vi "Create Reference.vi"(8 "error in (no error)":errorcluster, 11 "Generic":refnum<class "Generic.lvclass">) -> (0 "error out":errorcluster, 3 "Generic Reference":refnum<data-value>)   [LabVIEW 2013, in "Hierarchy Framework.lvlib" / "Generic.lvclass"]
doc: "Create class object data value reference."
uses:
  Generic.lvclass
panel:
  out "Generic Reference":u64
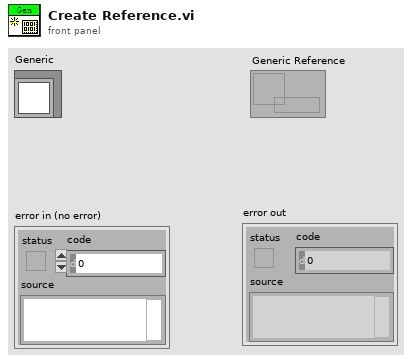
[diagram p1: front panel]
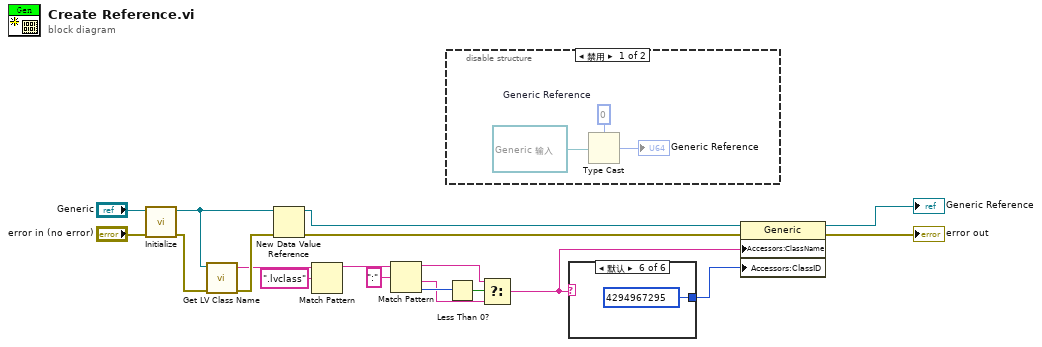
[diagram p0: block diagram]
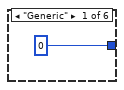
[diagram p3: hidden frame]
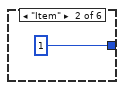
[diagram p4: hidden frame]
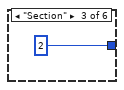
[diagram p5: hidden frame]
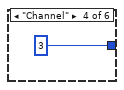
[diagram p6: hidden frame]
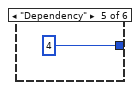
[diagram p7: hidden frame]
diagram:
  n1 = call-dynamic "Initialize.vi"("error in (no error)"="error in (no error)", "Generic输入"="Generic") -> ("error out"=w5:errorcluster, "Generic输出"=w7:refnum<class "Generic.lvclass">)  [unwired: 8 in]
  n2 = call <vilib>:"Get LV Class Name.vi"("error in (no error)"=w5, "object"=w7) -> ("error out"=w17:errorcluster, "class name"=w15:string)  [unwired: 8 in]
  n3 = New Data Value Reference(data value=w7, error in=w17) -> (data value reference=w3:refnum<data-value>, error out=w19:errorcluster)
  n4 = Match Pattern(string=w15, regular expression=".lvclass" ("class name")) -> (before substring=w13:string)  [unwired: 1 in, 3 out]
  n5 = Match Pattern(string=w13, regular expression=":" ("正则表达式")) -> (before substring=w1:string, after substring=w2:string, offset past match=w10:i32)  [unwired: 1 in, 1 out]
  n6 = disable-structure shown="禁用" {
    frame Disabled {
      w22 = u64 0  # Generic Reference
      n7 = Type Cast(type=w22, x=refnum<data-value> refnum ("Owner")) -> (*(type *) &x=→"Generic Reference":u64)
    }
    frame Enabled {
    }
  }
  n8 = Less Than 0?(x=w10) -> (x < 0?=w9:bool)
  n9 = Select(t=w1, s=w9, f=w2) -> (s? t:f=w8:string)
  n10 = case shown="默认" w8 {
    tunnel: [u32 0 ("ClassID") u32 1 ("ClassID") u32 2 ("ClassID") u32 3 ("ClassID") u32 4 ("ClassID") u32 4294967295 ("ClassID")] -> w14
    frame "Generic" {
    }
    frame "Item" {
    }
    frame "Section" {
    }
    frame "Channel" {
    }
    frame "Dependency" {
    }
    frame Default {
    }
  }
  n11 = property class="Generic"(reference=w3, error in=w19, "Accessors:ClassName"=w8, "Accessors:ClassID"=w14) -> (reference out=→"Generic Reference":refnum<data-value>, error out=→"error out":errorcluster)
